vi "GetMeasurementsHistory.vi"(7 "Base URL":string, 9 "Sensor":string, 10 "Limit":dbl, 11 "Device id":string) -> (0 "error out":errorcluster, 3 "Measurements":T1[](array[typedef]))   [LabVIEW 2026]
uses:
  MeasurementCluster.ctl
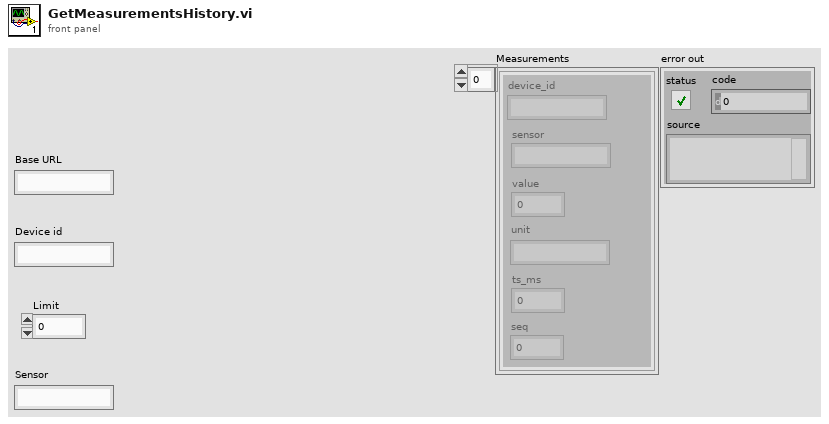
[diagram p1: front panel]
types:
  T1 = typedef "MeasurementCluster.ctl" = cluster{"device_id":string, "sensor":string, "value":dbl, "unit":string, "ts_ms":dbl, "seq":dbl}
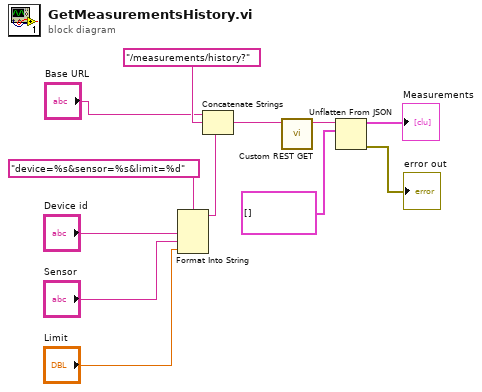
[diagram p0: block diagram]
diagram:
  n1 = Format Into String(format string="device=%s&sensor=%s&limit=%d", "Device id", "Sensor", "Limit") -> (resulting string=w8:string)  [unwired: 2 in, 1 out]
  n2 = Concatenate Strings("Base URL", "/measurements/history?" ("string"), w8) -> (w11:string)
  n3 = call "Custom REST GET.vi"("Base URL"=w11) -> ("body"=w12:string)  [unwired: 9 in, 1 out]
  n4 = Unflatten From JSON(JSON string=w12, type and defaults=T1[] []) -> (value=→"Measurements":T1[], error out=→"error out":errorcluster)  [unwired: 5 in]
